vi "Flush Read Buffer.vi"(8 "error in (no error)":errorcluster, 11 "VISA resource name":refnum<visa-resource-name>) -> (0 "error out":errorcluster, 3 "VISA resource name out":refnum<visa-resource-name>)   [LabVIEW 2017, in "JY-SPEX-TRIAX.lvlib"]
doc: "Flushes the read buffer by setting the timeout short, attempting to read 1024 bytes, and clearing any timeout error that may result. Useful for when a random message sometimes occurs and sometimes doesn't, messing up later reads."
uses:
  JY-SPEX-TRIAX.lvlib
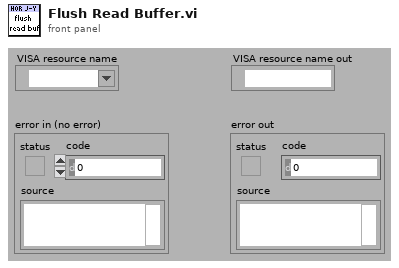
[diagram p1: front panel]
types:
  T1 = typedef "Semaphore RefNum" = refnum<k1>
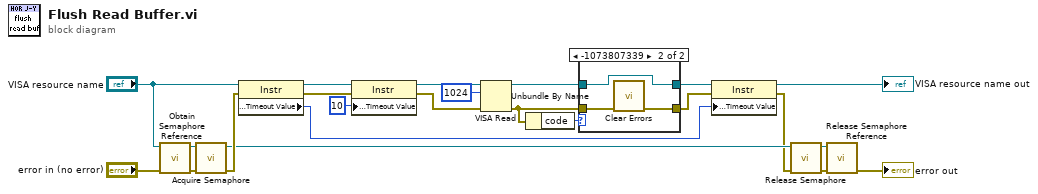
[diagram p0: block diagram]
diagram:
  n1 = call <vilib>:"Obtain Semaphore Reference.vi"("error in (no error)"="error in (no error)", "name (unnamed)"="VISA resource name") -> ("error out"=w10:errorcluster, "semaphore"=w9:T1)  [unwired: 1 in, 3 out]
  n2 = call <vilib>:"Acquire Semaphore.vi"("error in (no error)"=w10, "semaphore"=w9) -> ("error out"=w6:errorcluster, "semaphore out"=w3:T1)  [unwired: 1 in, 3 out]
  n3 = property class="Instr"(reference="VISA resource name", error in=w6) -> (reference out=w22:refnum<visa-resource-name>, error out=w21:errorcluster, "General Settings:Timeout Value"=w14:u32)
  n4 = property class="Instr"(reference=w22, error in=w21, "General Settings:Timeout Value"=u32 10) -> (reference out=w20:refnum<visa-resource-name>, error out=w19:errorcluster)
  n5 = VISA Read(VISA resource name=w20, byte count=u32 1024, error in (no error)=w19) -> (VISA resource name out=w15:refnum<visa-resource-name>, error out=w16:errorcluster)  [unwired: 2 out]
  n6 = Unbundle By Name(w16) -> ("code"=w17:i32)
  n7 = case shown="-1073807339" w17 {
    tunnel: w16 -> [w25 w28]
    tunnel: [w25 w27] -> w12
    tunnel: w15 -> [w24 w26]
    tunnel: [w24 w26] -> w13
    frame Default {
    }
    frame -1073807339 {
      n8 = call <vilib>:"Clear Errors.vi"("error in (no error)"=w28) -> ("error out"=w27:errorcluster)  [unwired: 1 in, 5 out]
    }
  }
  n9 = property class="Instr"(reference=w13, error in=w12, "General Settings:Timeout Value"=w14) -> (reference out=→"VISA resource name out":refnum<visa-resource-name>, error out=w2:errorcluster)
  n10 = call <vilib>:"Release Semaphore.vi"("error in (no error)"=w2, "semaphore"=w3) -> ("error out"=w5:errorcluster, "semaphore out"=w4:T1)  [unwired: 4 out]
  n11 = call <vilib>:"Release Semaphore Reference.vi"("error in (no error)"=w5, "semaphore"=w4) -> ("error out"=→"error out":errorcluster)  [unwired: 9 out]
